vi "Length_11.vi"() -> ()   [LabVIEW 2020]
uses:
  Support/Controls/Cmd_Mouse Popup.ctl
  Support/Controls/Clst_Initialize Input.ctl
  Support/Controls/Cmd_Var Data IO.ctl
  Variables/Global_Cal Info.vi
panel:
  out "기준기 분해능":string
  out "최소범위":string
  out "단위":string
  out "최대범위":string
  in  "Spec 변경":bool
  in  "Random":bool
  out "Spec":string[][](table)
  out "제목":string
  out "에러 출력":errorcluster
  out "Condition":string[][](table) caption="2. 직선성 시험"
  in  "Measured":string[][](table) caption="지시편차 (μm)"
  out "Load?":bool
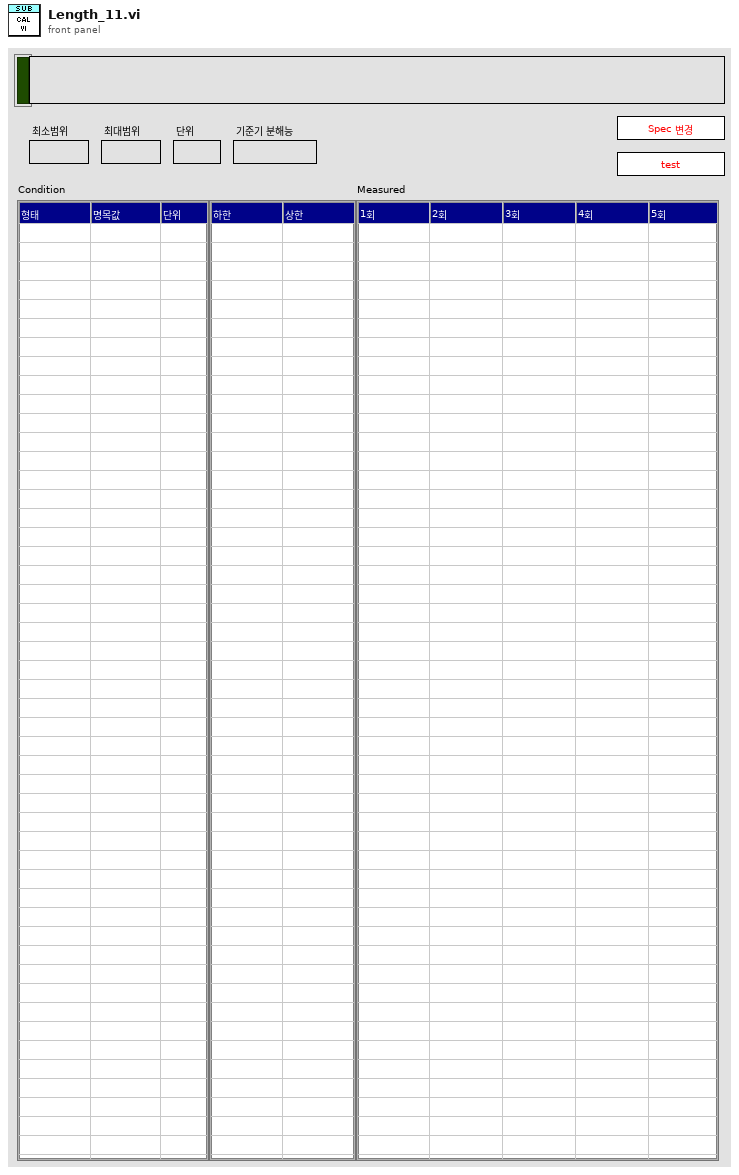
[diagram p1: front panel]
types:
  T1 = typedef "Cmd_Mouse Popup.ctl" = enum16{"활성화", "메뉴선택"}
  T2 = cluster{"Shift":bool, "Ctrl":bool, "Alt":bool, "Cmd":bool, "Opt":bool}
  T3 = typedef "Clst_Initialize Input.ctl" = cluster{"Initialize 1":cluster{"Condition":refnum<vi>[], "Spec":refnum<vi>[], "Measured":refnum<vi>[], "Resolution":refnum<vi>[], "Func_ext":string, "제목":refnum<vi>, "Measured_ADJ":refnum<vi>[]}, "Initialize 2":cluster{"문자열":refnum<vi>[], "콤보박스":refnum<vi>[], "링":refnum<vi>[], "열거형":refnum<vi>[], "테이블":refnum<vi>[], "여러열":refnum<vi>[], "디지털(DBL)":refnum<vi>[], "3D string":refnum<vi>[], "ctrl":refnum<vi>[], "boolean":refnum<vi>[]}}
  T4 = typedef "Cmd_Var Data IO.ctl" = enum16{"Condition", "Condition Default", "Condition_Temp", "Resolution", "Resolution Default", "Resolution Old", "Spec", "Spec Default", "Spec Old", "Spec Temp", "Result", "Result2", "Result3", "Result_Temp", "Result_ADJ", "Result_ADJ2", "STD1", "STD2", "STD3", "STD4", "STD5", "STD Temp", "CMC", "CMC Default"}
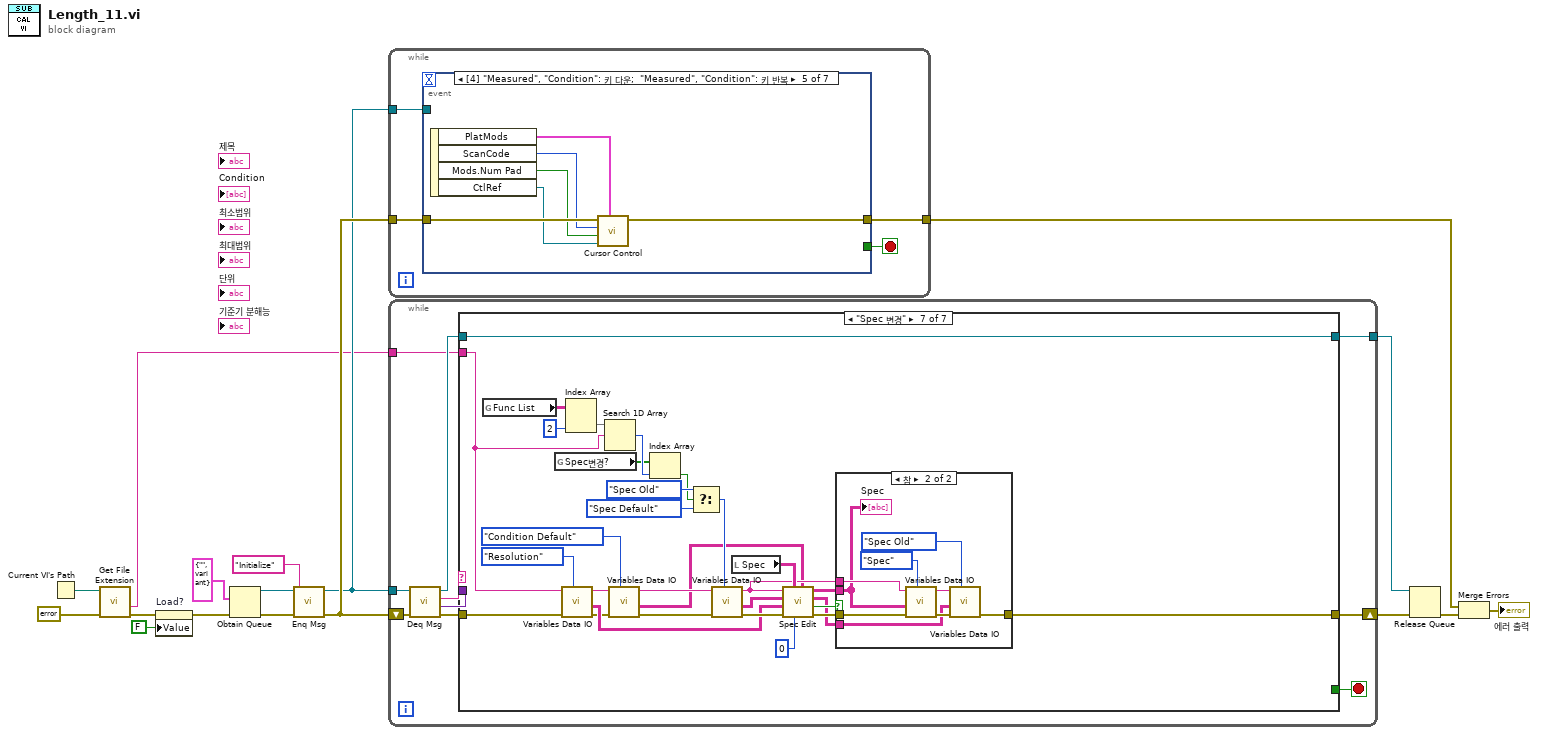
[diagram p0: block diagram]
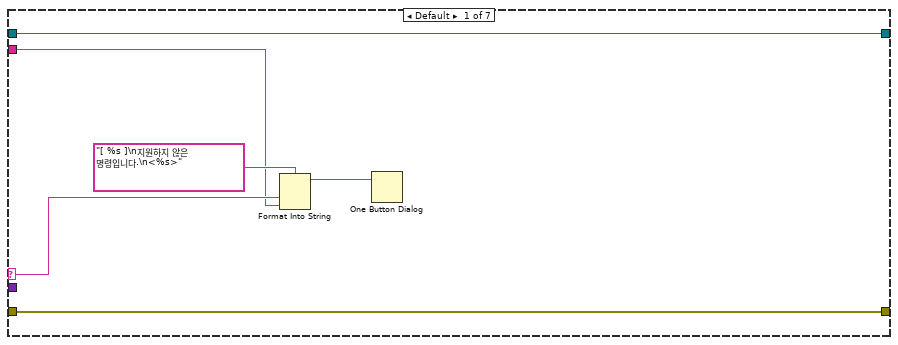
[diagram p2: hidden frame]
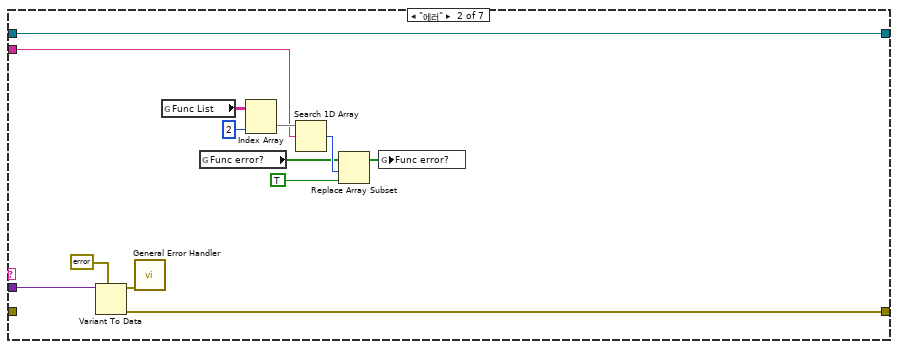
[diagram p3: hidden frame]
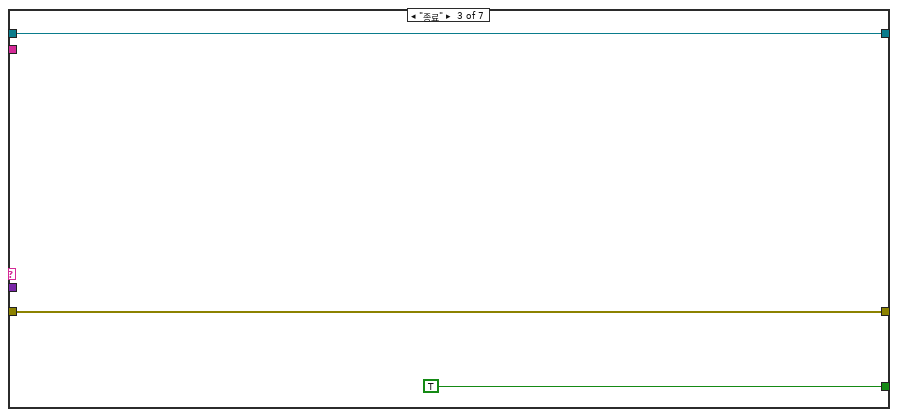
[diagram p4: hidden frame]
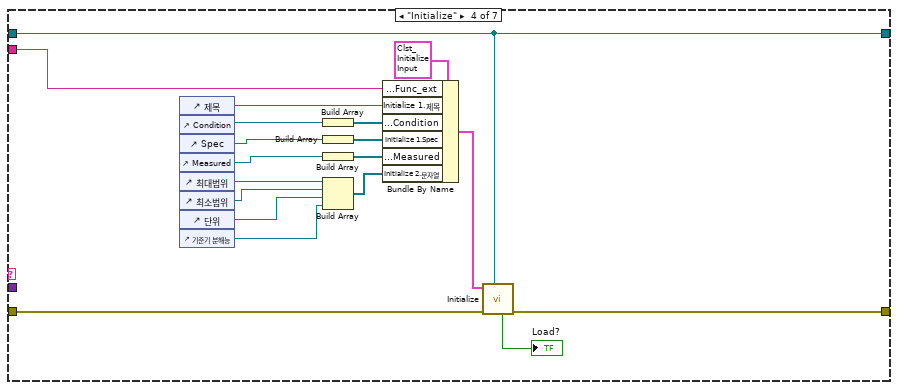
[diagram p5: hidden frame]
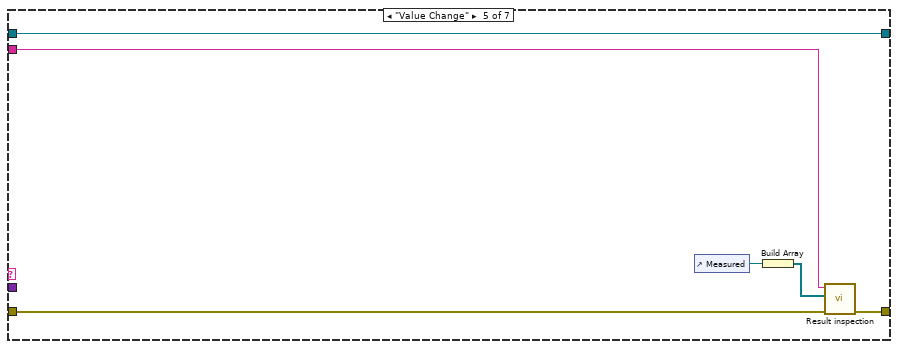
[diagram p6: hidden frame]
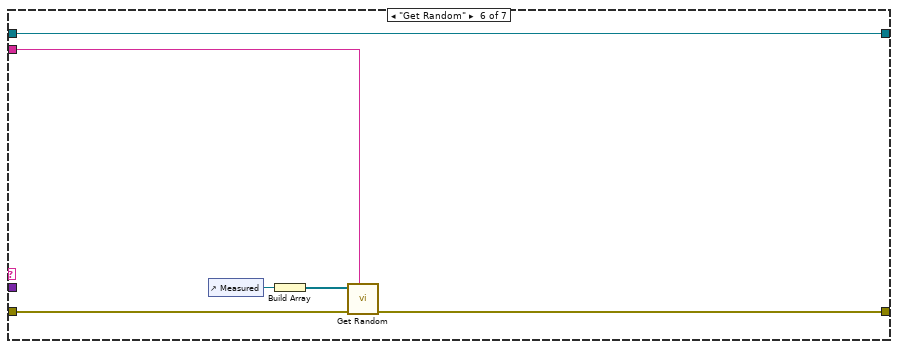
[diagram p7: hidden frame]
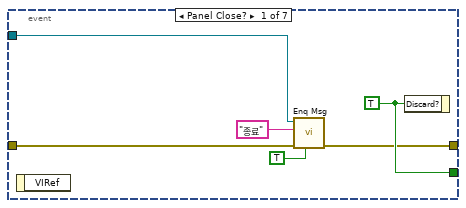
[diagram p9: hidden frame]
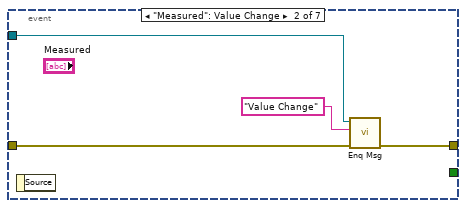
[diagram p10: hidden frame]
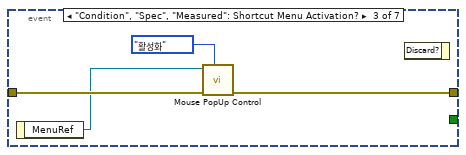
[diagram p11: hidden frame]
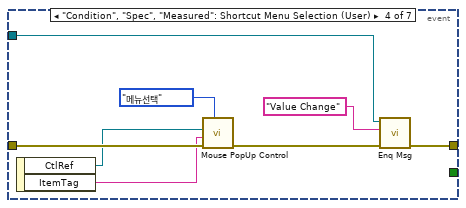
[diagram p12: hidden frame]
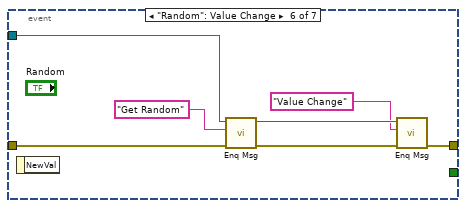
[diagram p13: hidden frame]
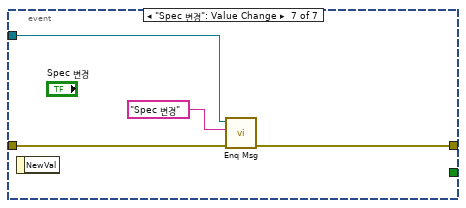
[diagram p14: hidden frame]
diagram:
  n1 = Current VI's Path() -> (path=w5:path)
  n2 = call <vilib>:"Get File Extension.vi"("error in (no error)"=errorcluster {"status"=FALSE, "code"=0, "source"=""} ("에러 상수"), "file"=w5) -> ("error out"=w3:errorcluster, "filename without extension"=w4:string)  [unwired: 5 in, 3 out]
  n3 = property on="Load?" class="Bool (엄격한)"(error in=w3, "Value"=FALSE ("Load?")) -> (error out=w2:errorcluster)  [unwired: 1 in, 1 out]
  n4 = Obtain Queue(element data type=cluster{"메세지":string, "값":variant} {"메세지"="", "값"=variant} ("Message Cluster"), error in (no error)=w2) -> (queue out=w14:refnum<queue>, error out=w16:errorcluster)  [unwired: 3 in, 1 out]
  n5 = call "Enq Msg.vi"("에러 입력(에러 없음)"=w16, "메세지"="Initialize", "큐 입력"=w14) -> ("에러 출력"=w15:errorcluster, "큐 출력"=w12:refnum<queue>)  [unwired: 7 in]
  n6 = while {
    tunnel: w15 -> [w19]
    tunnel: w12 -> [w20]
    tunnel: [w18] -> w9
    stop <- w21 stop-if-true
    n7 = event shown="[4] \"Measured\", \"Condition\": 키 다운;  \"Measured\", \"Condition\": 키 반복" {
      selector: _ -> [_ _ _ _ _ _ _]
      dyn-events: _ -> [_ _ _ _ _ _ _]
      timeout: _ -> [_ _ _ _ _ _ _]
      tunnel: [w27 _ _ _ _ _ _] -> w21
      tunnel: w20 -> [w25 w31 _ w36 _ w54 w58]
      tunnel: w19 -> [w26 w29 w35 w43 w49 w55 w59]
      tunnel: [w23 w30 w34 w37 w48 w50 w57] -> w18
      event Panel Close? {
        w27 = TRUE ("버림?")
        n8 = event-data() -> ()  [unwired: 1 in, 1 out]
        n9 = call "Enq Msg.vi"("우선순위 메시지?"=TRUE, "에러 입력(에러 없음)"=w26, "메세지"="종료", "큐 입력"=w25) -> ("에러 출력"=w23:errorcluster)  [unwired: 6 in, 1 out]
        n10 = event-data("Discard?"=w27) -> ()  [unwired: 1 in, 1 out]
      }
      event "Measured": Value Change {
        n11 = event-data() -> ()  [unwired: 1 in, 1 out]
        n12 = call "Enq Msg.vi"("에러 입력(에러 없음)"=w29, "메세지"="Value Change", "큐 입력"=w31) -> ("에러 출력"=w30:errorcluster)  [unwired: 7 in, 1 out]
      }
      event "Condition", "Spec", "Measured": Shortcut Menu Activation? {
        n13 = event-data() -> ("MenuRef"=w33:refnum<k9>)  [unwired: 1 in]
        n14 = call "Mouse PopUp Control.vi"("type"=Cmd_Mouse_Popup."활성화", "error in"=w35, "메뉴 참조"=w33) -> ("error out"=w34:errorcluster)  [unwired: 8 in]
        n15 = event-data() -> ()  [unwired: 2 in, 1 out]
      }
      event "Condition", "Spec", "Measured": Shortcut Menu Selection (User) {
        n16 = event-data() -> ("CtlRef"=w41:refnum<vi>, "ItemTag"=w40:string)  [unwired: 1 in]
        n17 = call "Mouse PopUp Control.vi"("type"=Cmd_Mouse_Popup."메뉴선택", "error in"=w43, "아이템 태그"=w40, "Tbl 참조 번호"=w41) -> ("error out"=w38:errorcluster)  [unwired: 7 in]
        n18 = call "Enq Msg.vi"("에러 입력(에러 없음)"=w38, "메세지"="Value Change", "큐 입력"=w36) -> ("에러 출력"=w37:errorcluster)  [unwired: 7 in, 1 out]
      }
      event "Measured", "Condition": Key Down; "Measured", "Condition": Key Repeat {
        n19 = event-data() -> ("PlatMods"=w44:T2, "ScanCode"=w47:i16, "Mods.Num Pad"=w46:bool, "CtlRef"=w45:refnum<vi>)  [unwired: 1 in]
        n20 = call "Cursor Control.vi"("플랫폼 조합키"=w44, "참조"=w45, "Num Pad"=w46, "ScanCode"=w47, "error in"=w49) -> ("error out"=w48:errorcluster)  [unwired: 5 in, 1 out]
      }
      event "Random": Value Change {
        n21 = event-data() -> ()  [unwired: 1 in, 1 out]
        n22 = call "Enq Msg.vi"("에러 입력(에러 없음)"=w55, "메세지"="Get Random", "큐 입력"=w54) -> ("에러 출력"=w53:errorcluster, "큐 출력"=w52:refnum<queue>)  [unwired: 7 in]
        n23 = call "Enq Msg.vi"("에러 입력(에러 없음)"=w53, "메세지"="Value Change", "큐 입력"=w52) -> ("에러 출력"=w50:errorcluster)  [unwired: 7 in, 1 out]
      }
      event "Spec 변경": Value Change {
        n24 = event-data() -> ()  [unwired: 1 in, 1 out]
        n25 = call "Enq Msg.vi"("에러 입력(에러 없음)"=w59, "메세지"="Spec 변경", "큐 입력"=w58) -> ("에러 출력"=w57:errorcluster)  [unwired: 7 in, 1 out]
      }
    }
  }
  n26 = while {
    shift-right: [w70] -> w11
    shift-left: w15 -> [w69]
    tunnel: w12 -> [w67]
    tunnel: [w62] -> w10
    tunnel: w4 -> [w61]
    stop <- w63 stop-if-true
    n27 = call "Deq Msg.vi"("에러 입력(에러 없음)"=w69, "큐 입력"=w67) -> ("에러 출력"=w68:errorcluster, "값"=w64:variant, "메세지"=w66:string, "큐 출력"=w65:refnum<queue>)  [unwired: 6 in]
    n28 = case shown="\"Spec 변경\"" w66 {
      selector: w66 -> [w72 _ _ _ _ _ _]
      tunnel: w68 -> [w76 _ w92 w111 w114 w119 w146]
      tunnel: [w76 w86 w92 w103 w116 w120 w149] -> w70
      tunnel: w65 -> [w75 w85 w90 w99 w117 w123 w153]
      tunnel: w64 -> [_ w87 _ _ _ _ _]
      tunnel: [_ _ TRUE ("버림?") _ _ _ _] -> w63
      tunnel: [w75 w85 w90 w99 w117 w123 w153] -> w62
      tunnel: w61 -> [w71 w77 _ w100 w115 w118 w131]
      frame Default {
        n29 = Format Into String(format string="[ %s ]\n지원하지 않은 명령입니다.\n<%s>" ("메시지"), w72, w71) -> (resulting string=w73:string)  [unwired: 2 in, 1 out]
        n30 = One Button Dialog(message=w73) -> ()  [unwired: 1 in, 1 out]
      }
      frame "에러" {
        n31 = Variant To Data(type=errorcluster {"status"=FALSE, "code"=0, "source"=""} ("에러 출력"), Variant=w87) -> (data=w89:errorcluster, error out=w86:errorcluster)  [unwired: 1 in]
        n32 = call <vilib>:"General Error Handler.vi"("error in (no error)"=w89) -> ()  [unwired: 10 in, 5 out]
        n33 = global read "Global_Cal Info.vi" "Func List"() -> (w79:string[][])
        n34 = global read "Global_Cal Info.vi" "Func error?"() -> (w82:bool[])
        n35 = Index Array(array=w79, index (col)=2 ("비활성화된 인덱스 (열)")) -> (element=w80:string[])  [unwired: 1 in]
        n36 = Search 1D Array(1D array=w80, element=w77) -> (index of element=w83:i32)  [unwired: 1 in]
        n37 = Replace Array Subset(array=w82, new element=TRUE ("새 원소/부분배열"), index=w83) -> (w84:bool[])
        n38 = global write "Global_Cal Info.vi" "Func error?"(w84) -> ()
      }
      frame "종료" {
      }
      frame "Initialize" {
        n39 = control-ref of="제목"() -> (w104:refnum<vi>)
        n40 = control-ref of="Condition"() -> (w108:refnum<vi>)
        n41 = control-ref of="Spec"() -> (w102:refnum<vi>)
        n42 = control-ref of="Measured"() -> (w105:refnum<vi>)
        n43 = control-ref of="최대범위"() -> (w97:refnum<vi>)
        n44 = control-ref of="최소범위"() -> (w96:refnum<vi>)
        n45 = control-ref of="단위"() -> (w95:refnum<vi>)
        n46 = control-ref of="기준기 분해능"() -> (w94:refnum<vi>)
        n47 = Build Array(w108) -> (w107:refnum<vi>[])
        n48 = Build Array(w102) -> (w101:refnum<vi>[])
        n49 = Build Array(w105) -> (w106:refnum<vi>[])
        n50 = Build Array(w97, w96, w95, w94) -> (w98:refnum<vi>[])
        n51 = Bundle By Name(cluster=T3 {"Initialize 1"={"Condition"=[], "Spec"=[], "Measured"=[], "Resolution"=[], "Func_ext"="", "제목"=refnum, "Measured_ADJ"=[]}, "Initialize 2"={"문자열"=[], "콤보박스"=[], "링"=[], "열거형"=[], "테이블"=[], "여러열"=[], "디지털(DBL)"=[], "3D string"=[], "ctrl"=[], "boolean"=[]}} ("입력 클러스터"), "Initialize 1.Func_ext"=w100, "Initialize 1.제목"=w104, "Initialize 1.Condition"=w107, "Initialize 1.Spec"=w101, "Initialize 1.Measured"=w106, "Initialize 2.문자열"=w98) -> (w109:T3)
        n52 = call "Initialize.vi"("큐 입력"=w99, "error in"=w111, "입력 클러스터"=w109) -> ("error out"=w103:errorcluster, "Load?"=→"Load?":bool)  [unwired: 5 in, 2 out]
      }
      frame "Value Change" {
        n53 = control-ref of="Measured"() -> (w113:refnum<vi>)
        n54 = Build Array(w113) -> (w112:refnum<vi>[])
        n55 = call "Result inspection.vi"("error in"=w114, "Ref. Data (Inspection)"=w112, "Func ext"=w115) -> ("error out"=w116:errorcluster)  [unwired: 5 in, 3 out]
      }
      frame "Get Random" {
        n56 = control-ref of="Measured"() -> (w122:refnum<vi>)
        n57 = Build Array(w122) -> (w121:refnum<vi>[])
        n58 = call "Get Random.vi"("Func_Ext"=w118, "에러 입력"=w119, "Meas"=w121) -> ("에러 출력"=w120:errorcluster)  [unwired: 7 in, 1 out]
      }
      frame "Spec 변경" {
        n59 = global read "Global_Cal Info.vi" "Func List"() -> (w136:string[][])
        n60 = global read "Global_Cal Info.vi" "Spec변경?"() -> (w132:bool[])
        n61 = call "Variables Data IO.vi"("Select"=Cmd_Var_Data_IO."Resolution", "error in"=w146, "Func_ext"=w131) -> ("error out"=w129:errorcluster, "Data Out"=w140:string[][], "Func_ext Out"=w127:string)  [unwired: 6 in]
        n62 = Index Array(array=w136, index (col)=2 ("비활성화된 인덱스 (열)")) -> (element=w134:string[])  [unwired: 1 in]
        n63 = Search 1D Array(1D array=w134, element=w131) -> (index of element=w133:i32)  [unwired: 1 in]
        n64 = call "Variables Data IO.vi"("Select"=Cmd_Var_Data_IO."Condition Default", "error in"=w129, "Func_ext"=w127) -> ("error out"=w128:errorcluster, "Data Out"=w124:string[][], "Func_ext Out"=w126:string)  [unwired: 6 in]
        n65 = Index Array(array=w132, index=w133) -> (element=w137:bool)
        n66 = Select(t=Cmd_Var_Data_IO."Spec Old" ("Select"), s=w137, f=Cmd_Var_Data_IO."Spec Default" ("Select")) -> (s? t:f=w130:T4)
        n67 = call "Variables Data IO.vi"("Select"=w130, "error in"=w128, "Func_ext"=w126) -> ("error out"=w148:errorcluster, "Data Out"=w141:string[][], "Func_ext Out"=w142:string)  [unwired: 6 in]
        n68 = local read "Spec"() -> (w143:string[][])
        n69 = call "Spec Edit.vi"("Condition"=w124, "열번호(기준값)"=0, "Spec Value"=w143, "에러 입력(에러 없음)"=w148, "Resolution"=w140, "Spec Default"=w141, "Func_ext"=w142) -> ("에러 출력"=w150:errorcluster, "변경?"=w151:bool, "Spec Default out"=w145:string[][], "Spec 출력"=w152:string[][])  [unwired: 1 in]
        n70 = case shown="참" w151 {
          tunnel: w152 -> [_ w160]
          tunnel: w150 -> [w154 w163]
          tunnel: [w154 w158] -> w149
          tunnel: w142 -> [_ w161]
          tunnel: w145 -> [_ w156]
          frame False {
          }
          frame True {
            n71 = call "Variables Data IO.vi"("Select"=Cmd_Var_Data_IO."Spec", "error in"=w163, "Data In"=w160, "Func_ext"=w161) -> ("error out"=w159:errorcluster, "Func_ext Out"=w157:string)  [unwired: 5 in, 1 out]
            n72 = call "Variables Data IO.vi"("Select"=Cmd_Var_Data_IO."Spec Old", "error in"=w159, "Data In"=w156, "Func_ext"=w157) -> ("error out"=w158:errorcluster)  [unwired: 5 in, 2 out]
            "Spec" <- w160
          }
        }
      }
    }
  }
  n73 = Release Queue(queue=w10, error in (no error)=w11) -> (error out=w8:errorcluster)  [unwired: 1 in, 2 out]
  n74 = Merge Errors(w9, w8) -> (→"에러 출력":errorcluster)
